vi "InitFrameBuffer.vi"() -> (0 "Init Data Out":fxp<+,3,3>[](array[numeric]))   [LabVIEW 2019, in "Initializers.lvlib"]
uses:
  Initializers.lvlib
panel:
  out "new picture":picture
  in  "path to PNG file":path=path "C:/Users/FreshBob/Dropbox/VIs/myRIO_GameConsole/Data/SplashScreen.png"
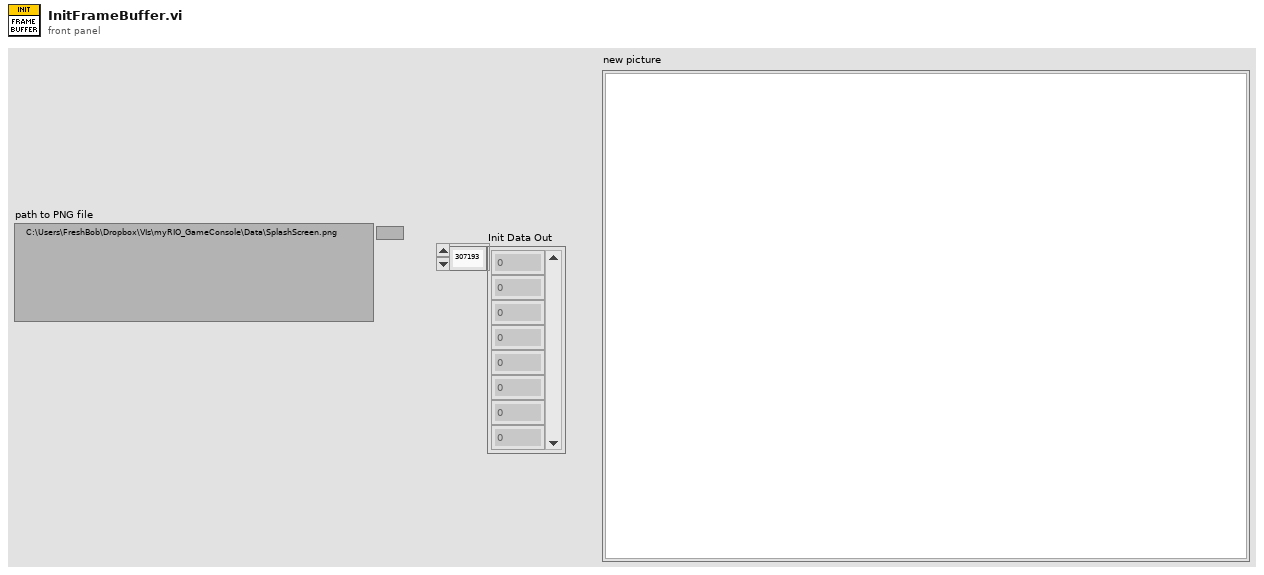
[diagram p1: front panel]
types:
  T1 = typedef "imagedata.ctl" = cluster{"image type":i32, "image depth":i32, "image":u8[], "mask":u8[], "colors":u32[], "Rectangle":cluster{"left":i16, "top":i16, "right":i16, "bottom":i16}}
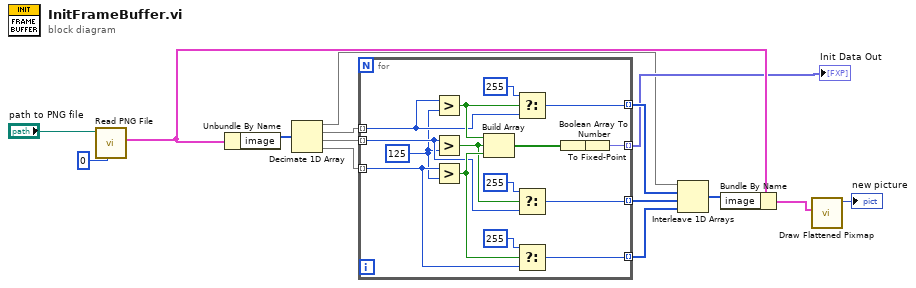
[diagram p0: block diagram]
diagram:
  n1 = call <vilib>:"Read PNG File.vi"("Transparency Thresh"=u8 0, "path to PNG file"="path to PNG file") -> ("image data"=w5:T1)  [unwired: 7 in, 2 out]
  n2 = Unbundle By Name(w5) -> ("image"=w10:u8[])
  n3 = Decimate 1D Array(w10) -> (w1:u8[], w11:u8[], w12:u8[], w13:u8[])
  n4 = for {
    tunnel: w11 -> [w21] mode=indexing
    tunnel: w12 -> [w25] mode=indexing
    tunnel: w13 -> [w24] mode=indexing
    tunnel: [w30] -> w4 mode=indexing
    tunnel: [w19] -> w8 mode=indexing
    tunnel: [w18] -> w7 mode=indexing
    tunnel: [w17] -> w6 mode=indexing
    w20 = u8 125 ("y")
    n5 = Greater?(x=w21, y=w20) -> (0:w29:bool)
    n6 = Greater?(x=w25, y=w20) -> (0:w27:bool)
    n7 = Greater?(x=w24, y=w20) -> (0:w28:bool)
    n8 = Build Array(w29, w27, w28) -> (w16:bool[])
    n9 = Select(t=u8 255, s=w29, f=w21) -> (s? t:f=w19:u8)
    n10 = Select(t=u8 255, s=w27, f=w25) -> (s? t:f=w18:u8)
    n11 = Select(t=u8 255, s=w28, f=w24) -> (s? t:f=w17:u8)
    n12 = Boolean Array To Number(Boolean array=w16) -> (number=w31:u32)
    n13 = To Fixed-Point(number=w31) -> (fixed-point=w30:fxp<+,3,3>)  [unwired: 1 in]
  }
  "Init Data Out" <- w4
  n14 = Interleave 1D Arrays(w1, w8, w7, w6) -> (w9:u8[])
  n15 = Bundle By Name(cluster=w5, "image"=w9) -> (w2:T1)
  n16 = call <vilib>:"Draw Flattened Pixmap.vi"("image data"=w2) -> ("new picture"=→"new picture":picture)  [unwired: 8 in]
